vi "Test Single Word.vi"() -> ()   [LabVIEW 2020]
uses:
  Wordle Engine.lvlib
panel:
  out "Results":string
  in  "Solver VI":path
  in  "Word to Test":string
  # "Instructions: Specify a Solver VI and a Word to Test and run the VI. The results of the solve will be displayed in the Results indicator."
  # "You can drag your solver VI into the path control before running to easily set the path."
  # "Leave blank to test a random word"
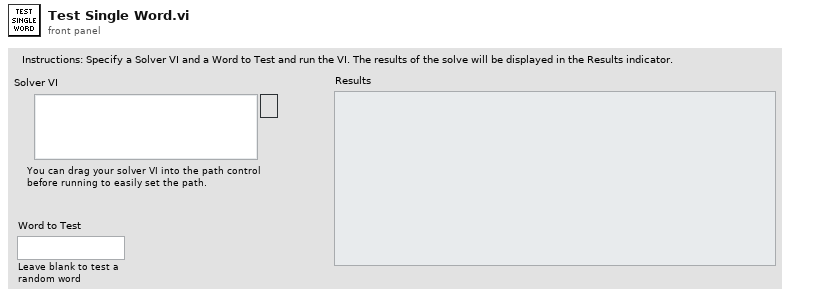
[diagram p1: front panel]
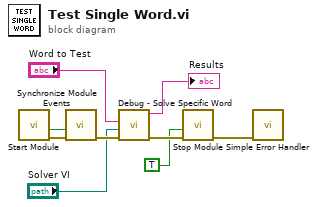
[diagram p0: block diagram]
diagram:
  n1 = call "Start Module.vi"() -> ("error out"=w9:errorcluster, "Wait for Event Sync?"=w8:bool)  [unwired: 8 in, 2 out]
  n2 = call "Synchronize Module Events.vi"("error in"=w9, "Wait for Event Sync?"=w8) -> ("error out"=w7:errorcluster)  [unwired: 9 in]
  n3 = call "Debug - Solve Specific Word.vi"("error in"=w7, "Solver VI"="Solver VI", "Word to Solve"="Word to Test") -> ("error out"=w3:errorcluster, "Results"=→"Results":string)  [unwired: 6 in, 1 out]
  n4 = call "Stop Module.vi"("error in"=w3, "Wait for Module to Stop? (F)"=TRUE) -> ("error out"=w1:errorcluster)  [unwired: 9 in]
  n5 = call <vilib>:"Simple Error Handler.vi"("error in (no error)"=w1) -> ()  [unwired: 4 in, 5 out]
